vi "Measurement Logic.vi"(8 "error in":errorcluster, 9 "measurement configuration":T2, 10 "measure call context in":refnum<class "Measure Call Context.lvclass">) -> (0 "error out":errorcluster, 1 "measurement results":T1={"Last SE Device"="Empty", "Last Route"=""}, 2 "measure call context out":refnum<class "Measure Call Context.lvclass">)   [LabVIEW 2025, in "Switch Executive Controller.lvclass"]
doc: "Contains the core logic for executing the measurement."
uses:
  Switch Executive Controller.lvclass
  <vilib>/Plug-In SDKs/Measurements/Measure Call Context/Measure Call Context.lvclass
  Measurement Configuration.ctl
  Measurement Results.ctl
  <vilib>/Plug-In SDKs/Clients/Session Management V1/Session Reservation/Session Reservation.lvclass/Session Reservation.ctl
  <vilib>/SwitchExecutive/nise.llb/niSE Multiconnect Mode Enum.ctl
  <vilib>/Plug-In SDKs/Clients/Session Management V1/Session Reservation/Get Session Info - 1Sess .vi
  <vilib>/Plug-In SDKs/Clients/Session Management V1/Session Reservation/Get Session Info - NSess .vi
  <vilib>/Plug-In SDKs/Clients/Session Management V1/Session Reservation/Merge Invalid DVR Error.vi
  <vilib>/Plug-In SDKs/Clients/Session Management V1/Session Reservation/Is DVR Valid.vi
  <vilib>/Plug-In SDKs/Measurements/Helpers/Error Strings Global Internal.vi
  <vilib>/Utility/error.llb/Error Cluster From Error Code.vi
  <extravilib>/ChannelInstances/Event Messenger-bool/Instantiate.vi
  <vilib>/Plug-In SDKs/Clients/Session Management V1/Session Reservation/Session Reservation.lvclass
  Switch Executive Controller.lvclass/Switch Executive Controller.ctl
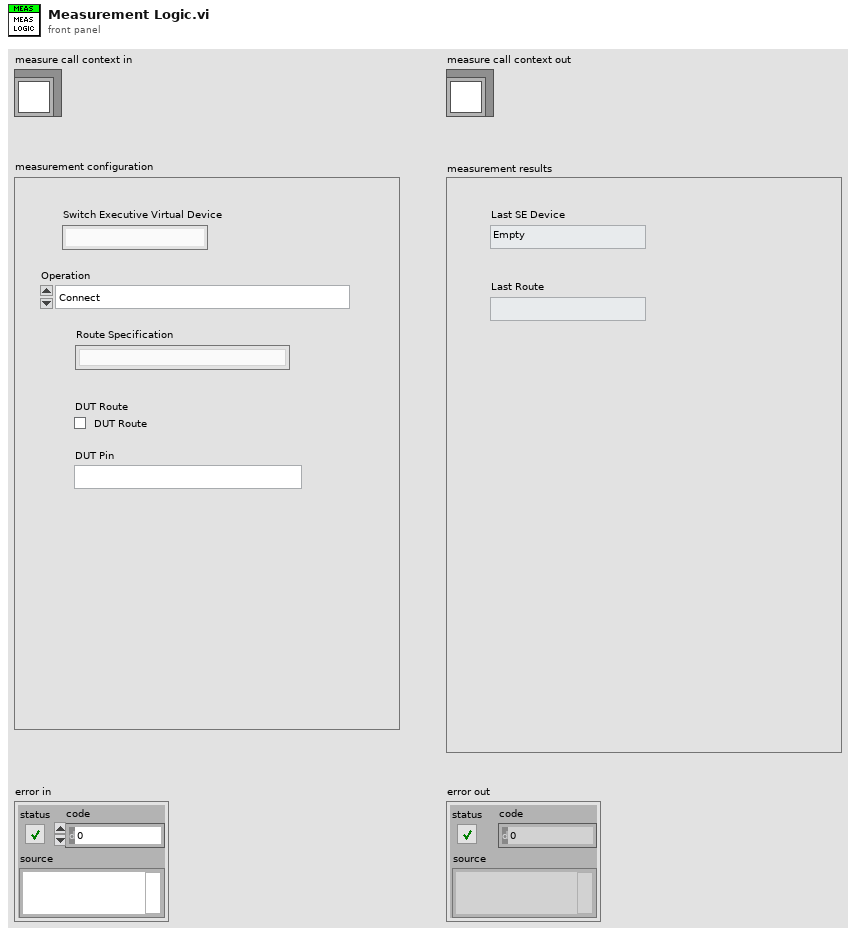
[diagram p1: front panel]
types:
  T1 = typedef "Switch Executive Controller.lvclass/Measurement Results.ctl" = cluster{"Last SE Device":string, "Last Route":string}
  T2 = typedef "Switch Executive Controller.lvclass/Measurement Configuration.ctl" = cluster{"Switch Executive Virtual Device":string, "Operation":enum32{"Connect", "Disconnect", "Disconnect All"}, "Route Specification":string, "DUT Pin":string, "DUT Route":bool}
  T3 = enum32{"Connect", "Disconnect", "Disconnect All"}
  T4 = typedef "ni.measurementlink.sessionmanagement.v1.api.lvlib/ni_measurementlink_sessionmanagement_v1_SessionInformation.ctl" = cluster{"session":T5, "resource_name":string, "channel_list":string, "instrument_type_id":string, "session_exists":bool, "session_reserved":bool, "channel_mappings":T6[], "annotations":T7[]}
  T5 = typedef "ni.measurementlink.sessionmanagement.v1.api.lvlib/nidevice_grpc_Session.ctl" = cluster{"name":string}
  T6 = typedef "ni.measurementlink.sessionmanagement.v1.api.lvlib/ni_measurementlink_sessionmanagement_v1_ChannelMapping.ctl" = cluster{"pin_or_relay_name":string, "site":i32, "channel":string, "multiplexer_resource_name":string, "multiplexer_route":string}
  T7 = typedef "ni.measurementlink.sessionmanagement.v1.api.lvlib/ni_measurementlink_sessionmanagement_v1_SessionInformation_AnnotationsEntry.ctl" = cluster{"key":string, "value":string}
  T8 = typedef "niSE SessionRefnum.ctl" = refnum<k1>
  T9 = typedef "niSE Multiconnect Mode Enum.ctl" = i32
  T10 = typedef "Event Messenger-bool.lvlib/))Channel.ctl" = refnum<queue>
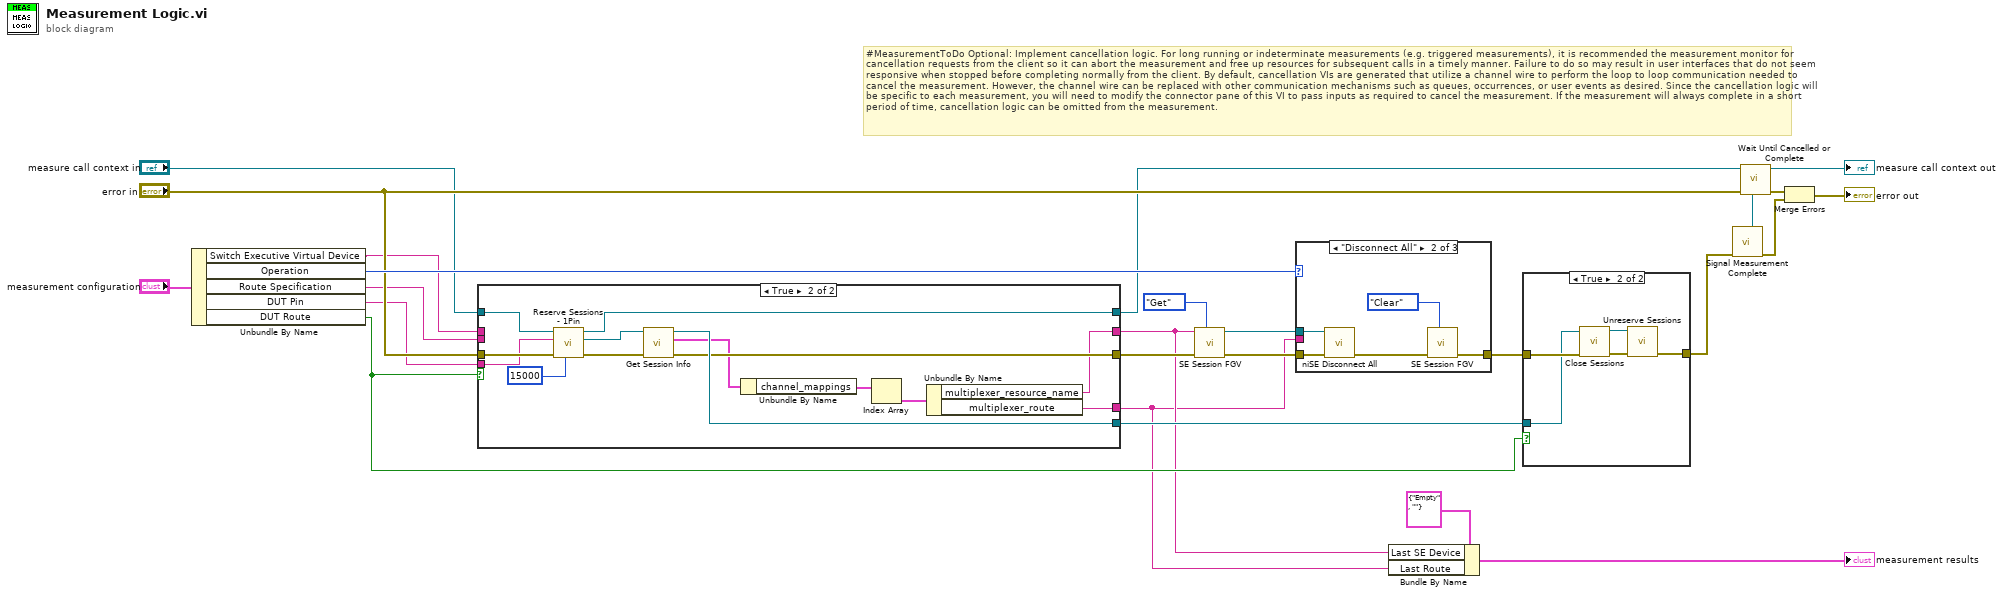
[diagram p0: block diagram]
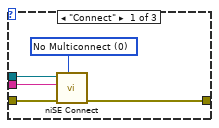
[diagram p3: hidden frame]
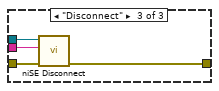
[diagram p4: hidden frame]
diagram:
  # "#MeasurementToDo Optional: Implement cancellation logic. For long running or indeterminate measurements (e.g. triggered measurements), it is recommended the measurement monitor for cancellation requests from the client so it can abort the measurement and free up resources for subsequent calls in a timely manner. Failure to do so may result in user interfaces that do not seem responsive when stopped before completing normally from the client. By default, cancellation VIs are generated that utilize a channel wire to perform the loop to loop communication needed to cancel the measurement. However, the channel wire can be replaced with other communication mechanisms such as queues, occurrences, or user events as desired. Since the cancellation logic will be specific to each measurement, you will need to modify the connector pane of this VI to pass inputs as required to cancel the measurement. If the measurement will always complete in a short period of time, cancellation logic can be omitted from the measurement."
  n1 = Unbundle By Name("measurement configuration") -> ("Switch Executive Virtual Device"=w9:string, "Operation"=w19:T3, "Route Specification"=w10:string, "DUT Pin"=w13:string, "DUT Route"=w11:bool)
  n2 = case shown="True" w11 {
    tunnel: "error in" -> [w29 w42]
    tunnel: "measure call context in" -> [w28 w41]
    tunnel: [_ w39] -> w14
    tunnel: [w29 w37] -> w8
    tunnel: w13 -> [_ w36]
    tunnel: [w28 w35] -> w12
    tunnel: w10 -> [w27 _]
    tunnel: [w27 w31] -> w2
    tunnel: [w26 w30] -> w3
    tunnel: w9 -> [w26 _]
    frame False {
    }
    frame True {
      n3 = call <vilib>:"Reserve Sessions - 1Pin.vi"("timeout (ms)"=15000 ("timeout in milliseconds"), "error in"=w42, "pin or relay name"=w36, "measurement context in"=w41) -> ("error out"=w38:errorcluster, "session reservation out"=w40:refnum<class "Session Reservation.lvclass">, "measurement context out"=w35:refnum<class "Measure Call Context.lvclass">)  [unwired: 5 in]
      n4 = call-poly <vilib>:"Get Session Info.vi"("error in"=w38, "session reservation in"=w40) -> ("error out"=w37:errorcluster, "session info"=w34:T4, "session reservation out"=w39:refnum<class "Session Reservation.lvclass">)  [unwired: 7 in]
      n5 = Unbundle By Name(w34) -> ("channel_mappings"=w33:T6[])
      n6 = Index Array(array=w33) -> (element=w32:T6)  [unwired: 1 in]
      n7 = Unbundle By Name(w32) -> ("multiplexer_resource_name"=w30:string, "multiplexer_route"=w31:string)
    }
  }
  n8 = call "SE Session FGV.vi"("Action"=enum16{"Get", "Clear"}."Get", "error in (no error)"=w8, "Virtual Device Name"=w3) -> ("error out"=w6:errorcluster, "NISE Session (out)"=w5:T8)  [unwired: 7 in]
  n9 = case shown="\"Disconnect All\"" w19 {
    tunnel: w5 -> [w48 w53 w57]
    tunnel: w6 -> [w47 w52 w56]
    tunnel: [w46 w50 w55] -> w18
    tunnel: w2 -> [w44 _ w54]
    frame "Connect" {
      w45 = T9 0 items=["Use Default Mode"=-1, "Multiconnect Routes"=1, "No Multiconnect"=0] ("Multiconnect Mode (Use Default Mode)")
      n10 = call <vilib>:"niSE Connect.vi"("Multiconnect Mode (Use Default Mode)"=w45, "error in (no error)"=w47, "Connection Specification (\"\")"=w44, "NISE Session (in)"=w48) -> ("error out"=w46:errorcluster)  [unwired: 6 in, 1 out]
    }
    frame "Disconnect All" {
      n11 = call <vilib>:"niSE Disconnect All.vi"("error in (no error)"=w52, "NISE Session (in)"=w53) -> ("error out"=w51:errorcluster)  [unwired: 4 in, 1 out]
      n12 = call "SE Session FGV.vi"("Action"=enum16{"Get", "Clear"}."Clear", "error in (no error)"=w51) -> ("error out"=w50:errorcluster)  [unwired: 8 in, 1 out]
    }
    frame "Disconnect" {
      n13 = call <vilib>:"niSE Disconnect.vi"("error in (no error)"=w56, "Disconnection Specification (\"\")"=w54, "NISE Session (in)"=w57) -> ("error out"=w55:errorcluster)  [unwired: 3 in, 1 out]
    }
  }
  n14 = Bundle By Name(cluster=T1 {"Last SE Device"="Empty", "Last Route"=""} ("measurement results"), "Last SE Device"=w3, "Last Route"=w2) -> (→"measurement results":T1)
  n15 = case shown="True" w11 {
    tunnel: w18 -> [w58 w61]
    tunnel: [w58 w60] -> w15
    tunnel: w14 -> [_ w59]
    frame False {
    }
    frame True {
      n16 = call <vilib>:"Close Sessions.vi"("error in"=w61, "session reservation in"=w59) -> ("error out"=w63:errorcluster, "session reservation out"=w62:refnum<class "Session Reservation.lvclass">)  [unwired: 8 in]
      n17 = call <vilib>:"Unreserve Sessions.vi"("error in"=w63, "session reservation in"=w62) -> ("error out"=w60:errorcluster)  [unwired: 9 in]
    }
  }
  n18 = call "Signal Measurement Complete.vi"("error in (no error)"=w15) -> ("error out"=w23:errorcluster, "done channel"=w24:T10)  [unwired: 9 in]
  n19 = call "Wait Until Cancelled or Complete.vi"("done channel"=w24, "error in (no error)"="error in", "measure call context in"=w12) -> ("error out"=w22:errorcluster, "measure call context out"=→"measure call context out":refnum<class "Measure Call Context.lvclass">)  [unwired: 7 in]
  n20 = Merge Errors(w22, w23) -> (→"error out":errorcluster)
